vi "Array to String Connected by Comma.vi"(7 "Split":string=",", 10 "State Queue":string, 11 "ColumnsList":string[](array[string])) -> (3 "Columns,String":string)   [LabVIEW 2021]
uses:
  <userlib>/sushu/sushu.lvlib
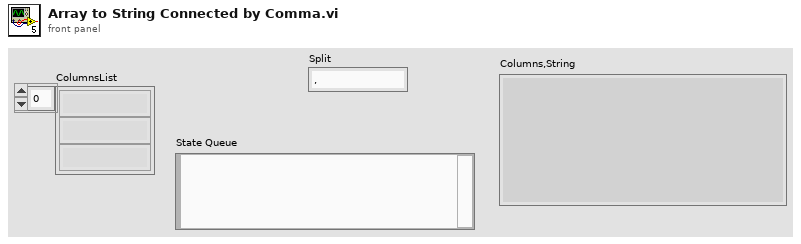
[diagram p1: front panel]
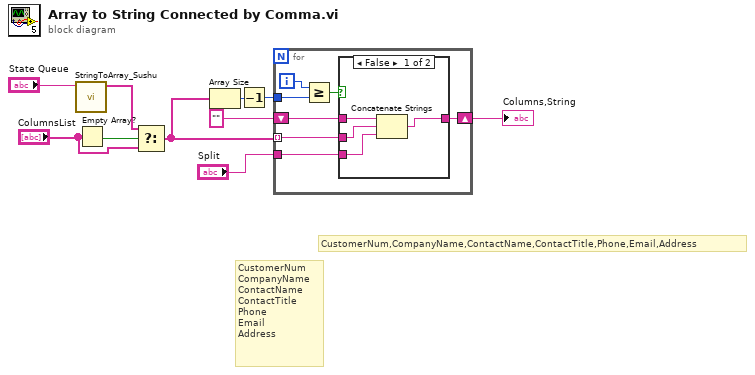
[diagram p0: block diagram]
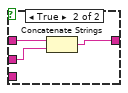
[diagram p2: hidden frame]
diagram:
  # "CustomerNum\nCompanyName\nContactName\nContactTitle\nPhone\nEmail\nAddress"
  # "CustomerNum,CompanyName,ContactName,ContactTitle,Phone,Email,Address"
  n1 = call <userlib>:"StringToArray_Sushu.vi"("State Queue"="State Queue") -> ("Array"=w7:string[])  [unwired: 7 in, 3 out]
  n2 = Empty Array?(array="ColumnsList") -> (empty?=w6:bool)
  n3 = Select(t=w7, s=w6, f="ColumnsList") -> (s? t:f=w9:string[])
  n4 = Array Size(array=w9) -> (size(s)=w2:i32)
  n5 = Decrement(x=w2) -> (x-1=w1:i32)
  n6 = for {
    tunnel: w9 -> [w14] mode=indexing
    shift-right: [w11] -> w5
    shift-left: "" -> [w12]
    tunnel: "Split" -> [w13]
    tunnel: w1 -> [w16]
    i -> [w17]
    n7 = Greater Or Equal?(x=w17, y=w16) -> (x >= y?=w15:bool)
    n8 = case shown="False" w15 {
      tunnel: w14 -> [w18 w22]
      tunnel: w13 -> [w21 _]
      tunnel: w12 -> [w20 w24]
      tunnel: [w19 w23] -> w11
      frame False {
        n9 = Concatenate Strings(w20, w18, w21) -> (w19:string)
      }
      frame True {
        n10 = Concatenate Strings(w24, w22) -> (w23:string)
      }
    }
  }
  "Columns,String" <- w5
